vi "Initialize OAuth for Salesforce.vi"(4 "Grant Flow (PKCE)":T1=enum."Authorization Code (PKCE)", 6 "Refresh Token":string, 9 "Salesforce Access Scope -- cluster":T2={"cdp_query_api"=FALSE, "pardot_api"=FALSE, "cdp_profile_api"=FALSE, "chatter_api"=FALSE, "cdp_ingest_api"=FALSE, "eclair_api"=FALSE, "wave_api"=FALSE, "api"=FALSE, "custom_permissions"=FALSE, "id"=FALSE, "profile"=TRUE, "email"=TRUE, "address"=FALSE, "phone"=FALSE, "lightning"=FALSE, "content"=FALSE, "openid"=TRUE, "full"=FALSE, "refresh_token"=TRUE, "offline_access"=FALSE, "visualforce"=FALSE, "web"=FALSE, "chatbot_api"=FALSE, "user_registration_api"=FALSE, "forgot_password"=FALSE, "cdp_api"=FALSE, "sfap_api"=FALSE, "interaction_api"=FALSE}, 10 "Client Secret":string, 11 "Client ID":string) -> (0 "error out":errorcluster, 3 "Oauth2.Salesforce.lvclass":refnum<class "Oauth2.Salesforce.lvclass">)   [LabVIEW 2017, in "Oauth2.Salesforce.lvclass"]
uses:
  Oauth2.Salesforce.lvclass
  D:/GitHub/Oauth2/source/Oauth2/Oauth2.lvclass
  Salesforce Access Scope -- cluster.ctl
  Oauth2/OAuth2 Flow -- enum.ctl
  Oauth2/Oauth2.lvclass
  <vilib>/LabVIEW Open Source Project/Data Manipulation/Variant/OpenVariant.lvlib
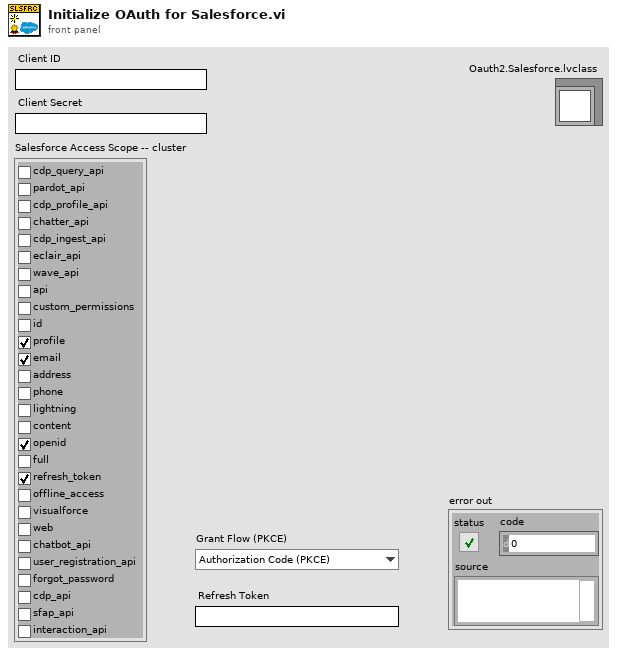
[diagram p1: front panel]
types:
  T1 = typedef "Oauth2.lvclass/OAuth2 Flow -- enum.ctl" = enum16{"Authorization Code", "Authorization Code (PKCE)", "Implicit", "Resource Owner Credentials", "Client Credentials"}
  T2 = typedef "Oauth2.Salesforce.lvclass/Salesforce Access Scope -- cluster.ctl" = cluster{"cdp_query_api":bool, "pardot_api":bool, "cdp_profile_api":bool, "chatter_api":bool, "cdp_ingest_api":bool, "eclair_api":bool, "wave_api":bool, "api":bool, "custom_permissions":bool, "id":bool, "profile":bool, "email":bool, "address":bool, "phone":bool, "lightning":bool, "content":bool, "openid":bool, "full":bool, "refresh_token":bool, "offline_access":bool, "visualforce":bool, "web":bool, "chatbot_api":bool, "user_registration_api":bool, "forgot_password":bool, "cdp_api":bool, "sfap_api":bool, "interaction_api":bool}
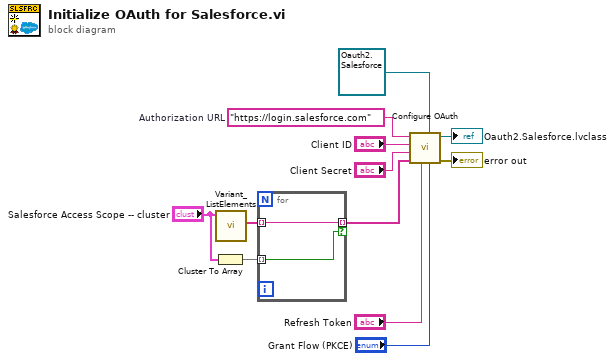
[diagram p0: block diagram]
diagram:
  w7 = "https://login.salesforce.com"  # Authorization URL
  n1 = Cluster To Array(cluster="Salesforce Access Scope -- cluster") -> (array=w4:bool[])
  n2 = call <vilib>:"Variant_ListElements.vi"("Variant"="Salesforce Access Scope -- cluster") -> ("element names"=w5:string[])  [unwired: 7 in, 3 out]
  n3 = for {
    tunnel: [w14] -> w2 mode=indexing if=w13
    tunnel: w5 -> [w14] mode=indexing
    tunnel: w4 -> [w13] mode=indexing
  }
  n4 = call "Configure OAuth.vi"("Grant Flow (PKCE)"="Grant Flow (PKCE)", "Oauth2 in"=refnum<class "Oauth2.Salesforce.lvclass"> refnum ("Oauth2.Google.lvclass"), "Refresh Token"="Refresh Token", "scopes"=w2, "Client Secret"="Client Secret", "Client ID"="Client ID", "Authorization Server URI"=w7) -> ("error out"=→"error out":errorcluster, "Oauth2"=→"Oauth2.Salesforce.lvclass":refnum<class "Oauth2.Salesforce.lvclass">)  [unwired: 3 in]
